vi "Example XYGraph Set BGK Color.vi"() -> ()   [LabVIEW 2015]
uses:
  <vilib>/ptbypt/NI_PtbyPt.lvlib
panel:
  in  "Color Box":u32(colorbox)
  out "XY Graph":cluster{dbl[], dbl[]}[](graph)
  # "Set any color here, the \ngrid lines will automatically\nbe adjusted for easy viewing"
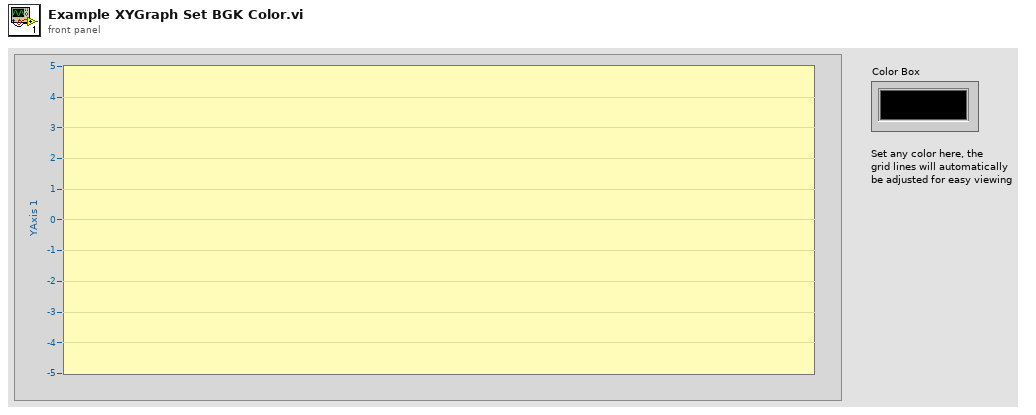
[diagram p1: front panel]
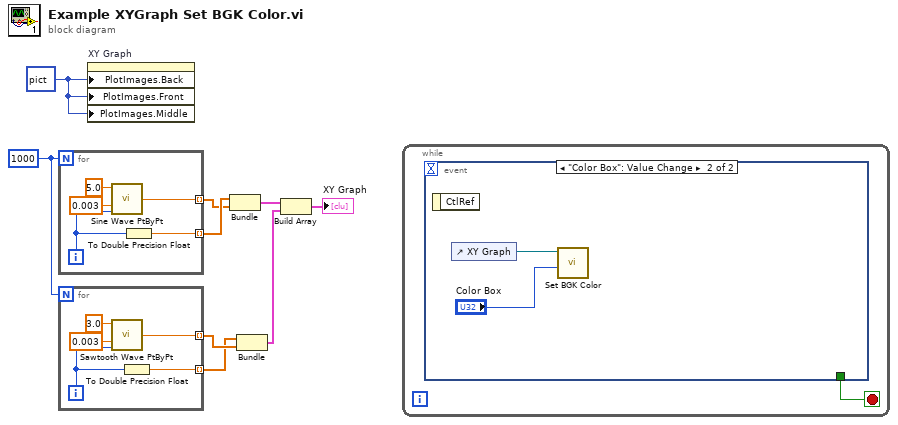
[diagram p0: block diagram]
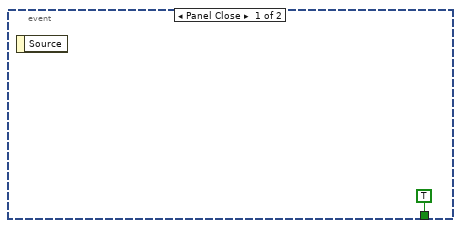
[diagram p2: hidden frame]
diagram:
  w1 = picture data[5B] ("Plot Images:Back")
  w2 = 1000
  n1 = for {
    N: w2 -> [_]
    tunnel: [w14] -> w8 mode=indexing
    tunnel: [w10] -> w9 mode=indexing
    i -> [w13]
    n2 = call <vilib>:"Sine Wave PtByPt.vi"("time"=w13, "frequency"=0.003, "amplitude"=5.0) -> ("sine wave"=w14:dbl)  [unwired: 1 in]
    n3 = To Double Precision Float(number=w13) -> (double precision float=w10:dbl)
  }
  n4 = for {
    N: w2 -> [_]
    tunnel: [w19] -> w5 mode=indexing
    tunnel: [w15] -> w4 mode=indexing
    i -> [w18]
    n5 = call <vilib>:"Sawtooth Wave PtByPt.vi"("time"=w18, "frequency"=0.003, "amplitude"=3.0) -> ("sawtooth wave"=w19:dbl)  [unwired: 1 in]
    n6 = To Double Precision Float(number=w18) -> (double precision float=w15:dbl)
  }
  n7 = property on="XY Graph" class="XYGraph (strict)"("PlotImages.Back"=w1, "PlotImages.Front"=w1, "PlotImages.Middle"=w1) -> ()  [unwired: 2 in, 2 out]
  n8 = Bundle(w9, w8) -> (w7:cluster{dbl[], dbl[]})  [unwired: 1 in]
  n9 = Bundle(w4, w5) -> (w3:cluster{dbl[], dbl[]})  [unwired: 1 in]
  n10 = Build Array(w7, w3) -> (→"XY Graph":cluster{dbl[], dbl[]}[])
  n11 = while {
    stop <- w20 stop-if-true
    n12 = event shown="[1] \"Color Box\": Value Change" {
      selector: _ -> [_ _]
      dyn-events: _ -> [_ _]
      timeout: _ -> [_ _]
      tunnel: [TRUE _] -> w20
      event Panel Close {
        n13 = event-data() -> ()  [unwired: 1 in, 1 out]
      }
      event "Color Box": Value Change {
        n14 = event-data() -> ()  [unwired: 1 in, 1 out]
        n15 = control-ref of="XY Graph"() -> (w22:refnum<vi>)
        n16 = call "Set BGK Color.vi"("color"="Color Box", "XYGraph"=w22) -> ()  [unwired: 8 in, 2 out]
      }
    }
  }
